vi "量程参数读取.vi"(8 "error in (no error)":errorcluster caption="错误输入（无错误）", 11 "测量参数":u16(ring) items=["COD"=22, "氨氮"=3, "总氮"=2, "总磷"=1]) -> (0 "error out":errorcluster caption="错误输出", 3 "量程参数读取":T1)   [LabVIEW 2016, in "斯坦道总磷.lvlib"]
uses:
  <vilib>/Plasmionique/MB Master/MB Master.lvlib
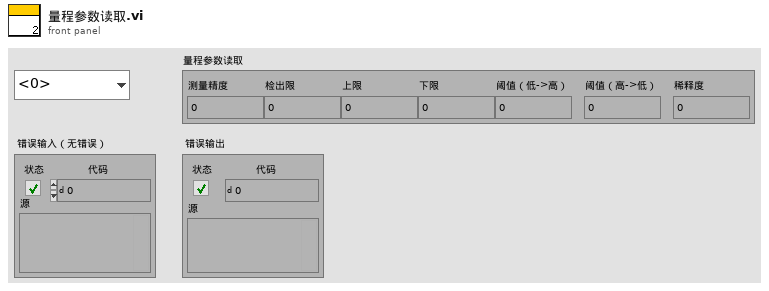
[diagram p1: front panel]
types:
  T1 = cluster{"测量精度":u16, "检出限":dbl, "上限":dbl, "下限":dbl, "阈值（低->高）":dbl, "阈值（高->低）":dbl, "稀释度":dbl}
  T2 = cluster{"FLOAT[0]":sgl, "FLOAT[1]":sgl, "FLOAT[2]":sgl, "FLOAT[3]":sgl, "FLOAT[4]":sgl}
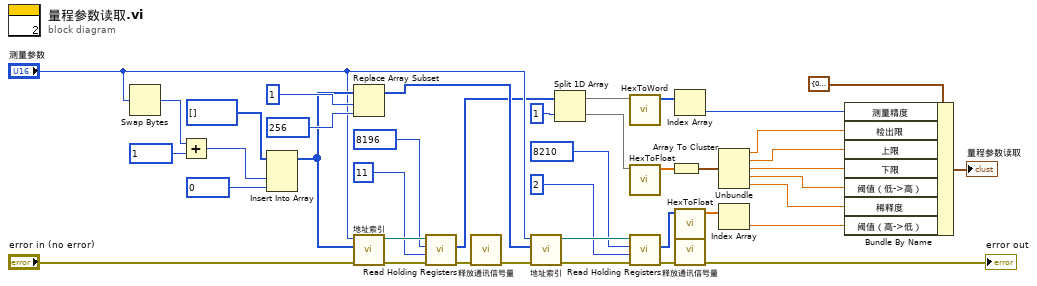
[diagram p0: block diagram]
diagram:
  n1 = Swap Bytes(anything="测量参数") -> (byte swapped=w19:u16)
  n2 = Add(x=w19, y=u16 1 ("starting address")) -> (x+y=w40:u16)
  n3 = Insert Into Array(array=u16[] [] ("数组"), new element #1=w40, new element #2=u16 0 ("starting address")) -> (w13:u16[])  [unwired: 1 in]
  n4 = Replace Array Subset(array=w13, new element=u16 256 ("starting address"), index=1 ("索引")) -> (w8:u16[])
  n5 = call "地址索引.vi"("error in (no error)"="error in (no error)", "values"=w13, "测量参数"="测量参数") -> ("error out"=w18:errorcluster, "MB session out"=w12:refnum<class "MB_Master.lvclass">)  [unwired: 7 in]
  n6 = call <vilib>:"Read Holding Registers.vi"("error in (no error)"=w18, "quantity"=u16 11, "starting address"=u16 8196, "MB session in"=w12) -> ("error out"=w17:errorcluster, "Registers"=w4:u16[])  [unwired: 5 in, 1 out]
  n7 = call "释放通讯信号量.vi"("error in (no error)"=w17) -> ("error out"=w14:errorcluster)  [unwired: 10 in]
  n8 = call "地址索引.vi"("error in (no error)"=w14, "values"=w8, "测量参数"="测量参数") -> ("error out"=w15:errorcluster, "MB session out"=w7:refnum<class "MB_Master.lvclass">)  [unwired: 7 in]
  n9 = Split 1D Array(array=w4, index=1 ("长度")) -> (first subarray=w26:u16[], second subarray=w25:u16[])
  n10 = call "HexToWord.vi"("数组"=w26) -> ("WORD"=w36:u16[])  [unwired: 10 in]
  n11 = call "HexToFloat.vi"("数组"=w25) -> ("FLOAT"=w41:sgl[])  [unwired: 10 in]
  n12 = call <vilib>:"Read Holding Registers.vi"("error in (no error)"=w15, "quantity"=u16 2, "starting address"=u16 8210, "MB session in"=w7) -> ("error out"=w16:errorcluster, "Registers"=w3:u16[])  [unwired: 5 in, 1 out]
  n13 = Array To Cluster(array=w41) -> (cluster=w34:T2)
  n14 = Index Array(array=w36) -> (element=w35:u16)  [unwired: 1 in]
  n15 = call "HexToFloat.vi"("数组"=w3) -> ("FLOAT"=w28:sgl[])  [unwired: 10 in]
  n16 = call "释放通讯信号量.vi"("error in (no error)"=w16) -> ("error out"=→"error out":errorcluster)  [unwired: 10 in]
  n17 = Unbundle(w34) -> ("FLOAT[0]"=w33:sgl, "FLOAT[1]"=w32:sgl, "FLOAT[2]"=w31:sgl, "FLOAT[3]"=w30:sgl, "FLOAT[4]"=w29:sgl)
  n18 = Index Array(array=w28) -> (element=w22:sgl)  [unwired: 1 in]
  n19 = Bundle By Name(cluster=T1 {"测量精度"=0, "检出限"=0.0, "上限"=0.0, "下限"=0.0, "阈值（低->高）"=0.0, "阈值（高->低）"=0.0, "稀释度"=0.0} ("量程参数读取"), "测量精度"=w35, "检出限"=w33, "上限"=w32, "下限"=w31, "阈值（低->高）"=w30, "稀释度"=w29, "阈值（高->低）"=w22) -> (→"量程参数读取":T1)
